vi "cvt_temp.vi"() -> ()   [LabVIEW 2022 SP3]
panel:
  in  "stop 2":bool
  in  "stop":bool
  in  "Tf":dbl
  out "Tc":dbl
  in  "Python version 2":string
  in  "module path 2":path
  in  "function name 2":string
  in  "function name":string
  in  "module path":path
  in  "Python version":string
  out "Tf":dbl
  in  "Tc":dbl
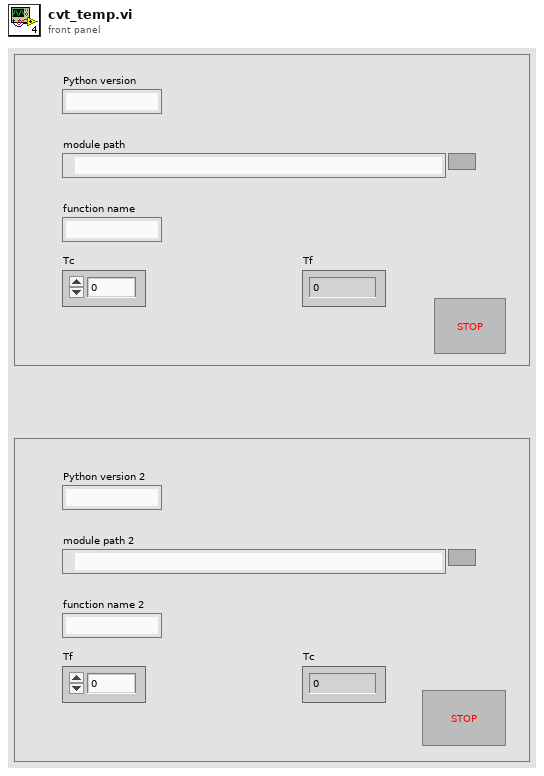
[diagram p1: front panel]
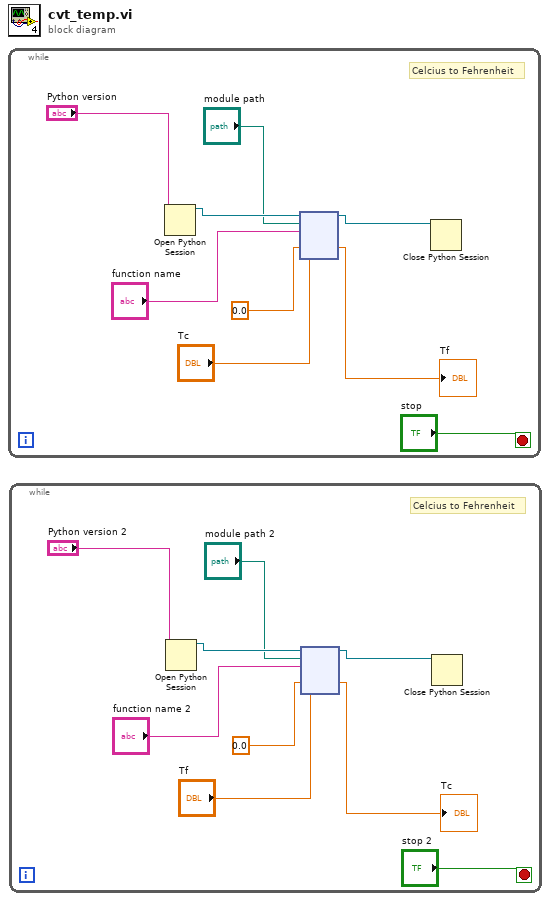
[diagram p0: block diagram]
diagram:
  n1 = while {
    stop <- "stop" stop-if-true
    # "Celcius to Fehrenheit"
    n2 = Open Python Session(python version="Python version") -> (session out=w8:refnum<k35>)  [unwired: 2 in, 1 out]
    n3 = node(w8, "module path", "function name", 0.0, "Tc") -> (w7:refnum<k35>, →"Tf":dbl)  [unwired: 2 in, 3 out]
    n4 = Close Python Session(session in=w7) -> ()  [unwired: 1 in, 1 out]
  }
  n5 = while {
    stop <- "stop 2" stop-if-true
    # "Celcius to Fehrenheit"
    n6 = Open Python Session(python version="Python version 2") -> (session out=w17:refnum<k35>)  [unwired: 2 in, 1 out]
    n7 = node(w17, "module path 2", "function name 2", 0.0, "Tf") -> (w16:refnum<k35>, →"Tc":dbl)  [unwired: 2 in, 3 out]
    n8 = Close Python Session(session in=w16) -> ()  [unwired: 1 in, 1 out]
  }
